vi "RFSG LO Signal Generation for 5668.vi"() -> ()   [LabVIEW 2017]
doc: "Demonstrates how to generate a sine wave at a specified frequency and power."
uses:
  <instrlib>/niRFSG/niRFSG.llb/niRFSG Ref Clock Sources.ctl
  <vilib>/Utility/error.llb/DialogType.ctl
panel:
  in  "Clock Source":T1="OnboardClock"
  in  "Resource Name":refnum<k15>="RFSG" caption="resource name"
  in  "Power Level (dBm)":dbl=-5.0 format="%_3f"
  in  "Frequency (Hz)":dbl=1000000000.0 format="%#.3p"
  in  "Stop":bool
  # "Overview: Demonstrates how to generate a sine wave at a specified frequency and power.\nRequirements: NI-RFSG\nInstructions:\n1. Change the Resource Name to your device.\n2. Run the VI.\n3. Click Stop to stop the VI."
  # "In order to configure new settings you must stop the example using the Stop button and then run the example with the new settings."
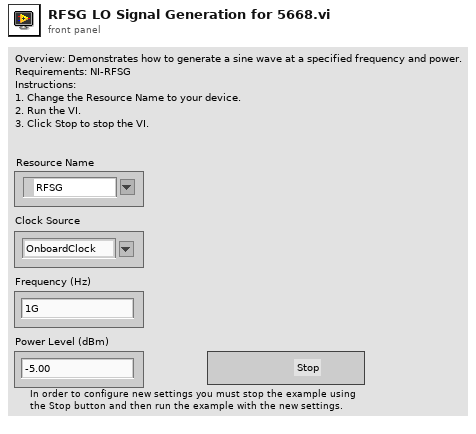
[diagram p1: front panel]
types:
  T1 = typedef "niRFSG Ref Clock Sources.ctl" = string
  T2 = typedef "DialogType.ctl" = u16
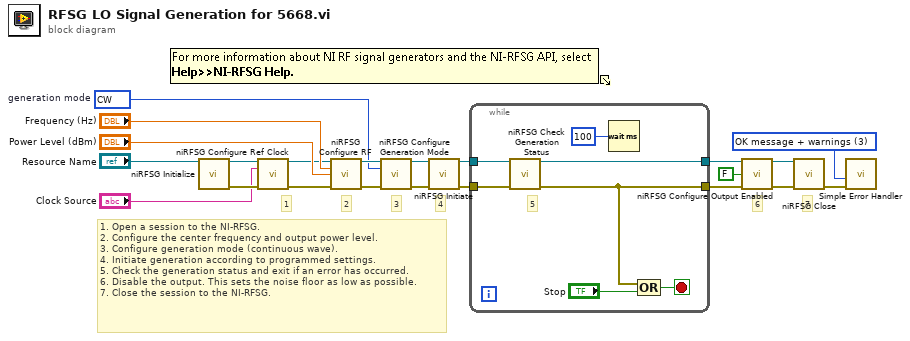
[diagram p0: block diagram]
diagram:
  w2 = T2 3 items=["no dialog", "OK message", "continue or stop message", "OK message + warnings", "continue/stop + warnings"] ("type of dialog (OK msg:1)")
  w12 = 1000 items=["CW"=1000, "Arb Waveform"=1001, "Script"=1002]  # generation mode
  # "3"
  # "6"
  # "7"
  # "4"
  # "2"
  # "1"
  # "1. Open a session to the NI-RFSG.\n2. Configure the center frequency and output power level.\n3. Configure generation mode (continuous wave).\n4. Initiate generation according to programmed settings.\n5. Check the generation status and exit if an error has occurred.\n6. Disable the output. This sets the noise floor as low as possible.\n7. Close the session to the NI-RFSG."
  n1 = call <instrlib>:"niRFSG Initialize.vi"("resource name"="Resource Name") -> ("instrument handle"=w22:refnum<k15>, "error out"=w7:errorcluster)  [unwired: 13 in]
  n2 = call <instrlib>:"niRFSG Configure Ref Clock.vi"("instrument handle"=w22, "ref clock source"="Clock Source", "error in"=w7) -> ("instrument handle out"=w8:refnum<k15>, "error out"=w6:errorcluster)  [unwired: 11 in]
  n3 = call <instrlib>:"niRFSG Configure RF.vi"("instrument handle"=w8, "frequency (Hz)"="Frequency (Hz)", "power level (dBm)"="Power Level (dBm)", "error in"=w6) -> ("instrument handle out"=w13:refnum<k15>, "error out"=w16:errorcluster)  [unwired: 10 in]
  n4 = call <instrlib>:"niRFSG Configure Generation Mode.vi"("instrument handle"=w13, "generation mode"=w12, "error in"=w16) -> ("instrument handle out"=w14:refnum<k15>, "error out"=w15:errorcluster)  [unwired: 11 in]
  n5 = call <instrlib>:"niRFSG Initiate.vi"("instrument handle"=w14, "error in"=w15) -> ("instrument handle out"=w21:refnum<k15>, "error out"=w3:errorcluster)  [unwired: 12 in]
  n6 = while {
    tunnel: w21 -> [w25]
    tunnel: [w26] -> w17
    tunnel: [w24] -> w4
    tunnel: w3 -> [w23]
    stop <- w29 stop-if-true
    # "5"
    n7 = call <instrlib>:"niRFSG Check Generation Status.vi"("instrument handle"=w25, "error in"=w23) -> ("instrument handle out"=w26:refnum<k15>, "error out"=w24:errorcluster)  [unwired: 11 in, 1 out]
    n8 = Wait (ms)(milliseconds to wait=u32 100) -> ()  [unwired: 1 out]
    n9 = Compound Arithmetic op=OR(w24, "Stop") -> (w29:bool)
  }
  n10 = call <instrlib>:"niRFSG Configure Output Enabled.vi"("instrument handle"=w17, "output enabled"=FALSE ("output enable"), "error in"=w4) -> ("instrument handle out"=w20:refnum<k15>, "error out"=w19:errorcluster)  [unwired: 11 in]
  n11 = call <instrlib>:"niRFSG Close.vi"("instrument handle"=w20, "error in"=w19) -> ("error out"=w1:errorcluster)  [unwired: 13 in]
  n12 = call <vilib>:"Simple Error Handler.vi"("type of dialog (OK msg:1)"=w2, "error in (no error)"=w1) -> ()  [unwired: 3 in, 5 out]
